vi "Acquire Triggered Images.vi"() -> ()   [LabVIEW 2023]
doc: "The Acquire Triggered Image example acquires images continuously and displays the images in an image control. This VI demonstrates how to configure a triggered acquisition using a grab."
uses:
  <vilib>/vision/driver/IMAQdx.llb/IMAQdx Buffer Number Mode.ctl
  <vilib>/vision/driver/NI_Vision_Acquisition_Software.lvlib
  <resource>/objmgr/imaqdx.rc
panel:
  out "Trigger Rate":dbl
  in  "Simulated Processing Delay (ms)":i32
  out "Images Behind":i32
  in  "Trigger Parameters":T1={"Trigger Mode"=0, "Trigger Activation"=0, "Timeout (ms)"=1000} {"Trigger Activation" items=["Rising Edge", "Falling Edge"]; "Trigger Mode" items=["Off", "On"]}
  in  "Camera Name":refnum<k21> caption="IMAQdx Session"
  out "Missed Trigger":bool
  out "Buffer Number":u32
  out "Image":T2(plugin-control)
  in  "Stop":bool
  # "Overview: Demonstrates how to dynamically enumerate the trigger modes and configure a triggered acquisition.\nRequirements: Vision Acquisition Software\nInstructions: \n1. Select the Camera Name\n2. Run the VI\n3. Select a Trigger Mode\n4. Specify a Timeout\n5. Increase the Simulated Processing Delay to see the effect on the Images Behind when the acquisition loop isn't executed as quickly as the camera acquires images."
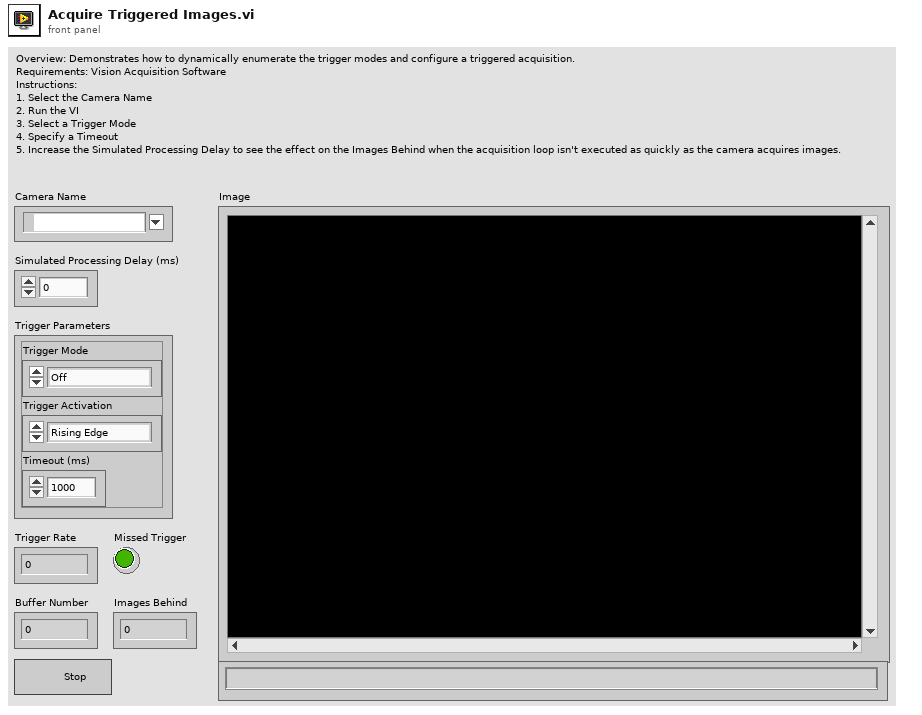
[diagram p1: front panel]
types:
  T1 = cluster{"Trigger Mode":u32, "Trigger Activation":u32, "Timeout (ms)":u32}
  T2 = typedef "IMAQ Image.ctl" = refnum<image>
  T3 = typedef "IMAQdx.ctl" = refnum<k21>
  T4 = typedef "NI_Vision_Acquisition_Software.lvlib/IMAQdx Buffer Number Mode.ctl" = enum32{"Next", "Last", "Buffer Number", "Every", "Last New"}
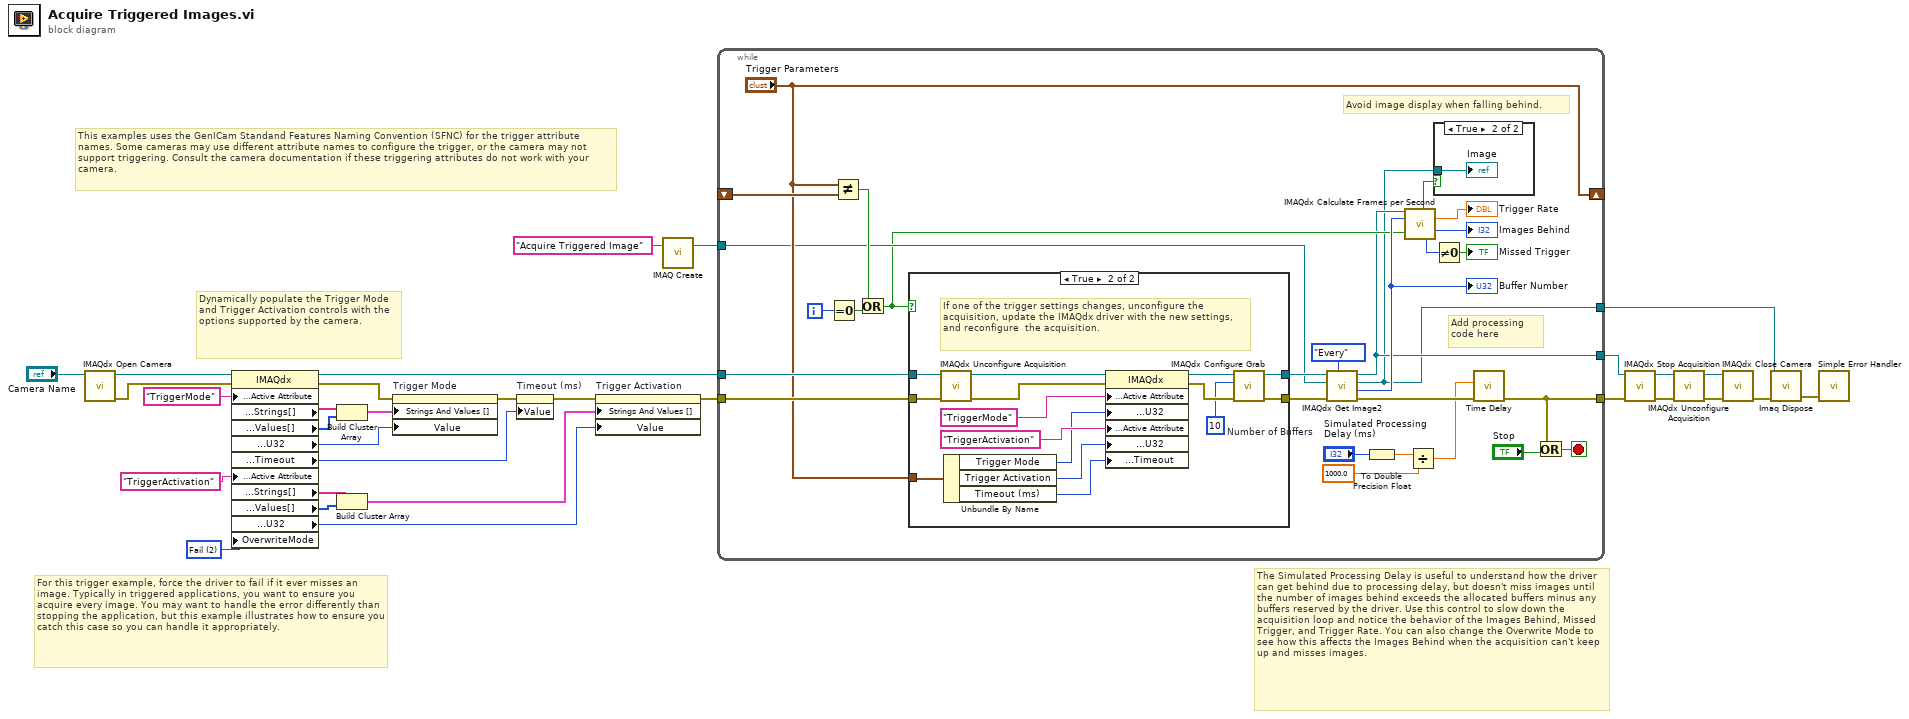
[diagram p0: block diagram]
diagram:
  w8 = u32 2 items=["Get Oldest"=0, "Fail"=2, "Get Newest"=3] ("OverwriteMode")
  # "The Simulated Processing Delay is useful to understand how the driver can get behind due to processing delay, but doesn't miss images until the number of images behind exceeds the allocated buffers minus any buffers reserved by the driver. Use this control to slow down the acquisition loop and notice the behavior of the Images Behind, Missed Trigger, and Trigger Rate. You can also change the Overwrite Mode to see how this affects the Images Behind when the acquisition can't keep up and misses images."
  # "For this trigger example, force the driver to fail if it ever misses an image. Typically in triggered applications, you want to ensure you acquire every image. You may want to handle the error differently than stopping the application, but this example illustrates how to ensure you catch this case so you can handle it appropriately."
  # "This examples uses the GenICam Standand Features Naming Convention (SFNC) for the trigger attribute names. Some cameras may use different attribute names to configure the trigger, or the camera may not support triggering. Consult the camera documentation if these triggering attributes do not work with your camera."
  # "Dynamically populate the Trigger Mode and Trigger Activation controls with the options supported by the camera."
  n1 = call <vilib>:"IMAQdx Open Camera.vi"("Session In"="Camera Name") -> ("error out"=w30:errorcluster, "Session Out"=w31:T3)  [unwired: 2 in, 7 out]
  n2 = property class="IMAQdx"(reference=w31, error in=w30, "Camera Attributes:Active Attribute"="TriggerMode" ("ActiveAttribute"), "Camera Attributes:Active Attribute"="TriggerActivation" ("ActiveAttribute"), "OverwriteMode"=w8) -> (reference out=w23:T3, error out=w25:errorcluster, "Camera Attributes:Enum:Strings[]"=w17:string[], "Camera Attributes:Enum:Values[]"=w16:u32[], "Camera Attributes:Value:U32"=w19:u32, "Acquisition Attributes:Timeout"=w22:u32, "Camera Attributes:Enum:Strings[]"=w14:string[], "Camera Attributes:Enum:Values[]"=w13:u32[], "Camera Attributes:Value:U32"=w18:u32)
  n3 = Build Cluster Array(w17, w16) -> (w15:cluster{string, u32}[])
  n4 = Build Cluster Array(w14, w13) -> (w12:cluster{string, u32}[])
  n5 = property on="Trigger Mode" class="Ring (strict)"(error in=w25, "Strings And Values []"=w15, "Value"=w19) -> (error out=w21:errorcluster)  [unwired: 1 in, 1 out]
  n6 = property on="Timeout (ms)" class="DigNum (strict)"(error in=w21, "Value"=w22) -> (error out=w20:errorcluster)  [unwired: 1 in, 1 out]
  n7 = property on="Trigger Activation" class="Ring (strict)"(error in=w20, "Strings And Values []"=w12, "Value"=w18) -> (error out=w24:errorcluster)  [unwired: 1 in, 1 out]
  n8 = call "IMAQ Create"("Image Name"="Acquire Triggered Image") -> ("New Image"=w27:T2)  [unwired: 3 in, 2 out]
  n9 = while {
    tunnel: [w44] -> w2
    tunnel: w23 -> [w57]
    tunnel: [w40] -> w3
    tunnel: w27 -> [w48]
    tunnel: w24 -> [w56]
    shift-right: ["Trigger Parameters"] -> _
    shift-left: _ -> [w55]
    tunnel: [w33] -> w10
    i -> [w54]
    stop <- w59 stop-if-true
    # "Avoid image display when falling behind."
    # "Add processing code here"
    n10 = Equal To 0?(x=w54) -> (x = 0?=w53:bool)
    n11 = Not Equal?(x="Trigger Parameters", y=w55) -> (x != y?=w52:bool)
    n12 = Or(x=w52, y=w53) -> (x .or. y?=w45:bool)
    n13 = case shown="True" w45 {
      tunnel: w57 -> [w62 w77]
      tunnel: [w62 w75] -> w50
      tunnel: w56 -> [w61 w76]
      tunnel: [w61 w74] -> w49
      tunnel: "Trigger Parameters" -> [_ w73]
      frame False {
      }
      frame True {
        w63 = u32 10  # Number of Buffers
        # "If one of the trigger settings changes, unconfigure the acquisition, update the IMAQdx driver with the new settings, and reconfigure  the acquisition."
        n14 = call <vilib>:"IMAQdx Unconfigure Acquisition.vi"("error in"=w76, "Session In"=w77) -> ("error out"=w71:errorcluster, "Session Out"=w72:T3)  [unwired: 8 out]
        n15 = Unbundle By Name(w73) -> ("Trigger Mode"=w66:u32, "Trigger Activation"=w65:u32, "Timeout (ms)"=w64:u32)
        n16 = property class="IMAQdx"(reference=w72, error in=w71, "Camera Attributes:Active Attribute"="TriggerMode" ("ActiveAttribute"), "Camera Attributes:Value:U32"=w66, "Camera Attributes:Active Attribute"="TriggerActivation" ("ActiveAttribute"), "Camera Attributes:Value:U32"=w65, "Acquisition Attributes:Timeout"=w64) -> (reference out=w70:T3, error out=w69:errorcluster)
        n17 = call <vilib>:"IMAQdx Configure Grab.vi"("error in"=w69, "Number of Buffers"=w63, "Session In"=w70) -> ("error out"=w74:errorcluster, "Session Out"=w75:T3)  [unwired: 7 out]
      }
    }
    n18 = call <vilib>:"IMAQdx Get Image2.vi"("Buffer Number Mode (Next)"=IMAQdx_Buffer_Number_Mode."Every", "error in"=w49, "Image In"=w48, "Session In"=w50) -> ("error out"=w41:errorcluster, "Buffer Number Out"=w46:u32, "Image Out"=w33:T2, "Session Out"=w44:T3)  [unwired: 4 in]
    "Buffer Number" <- w46
    n19 = To Double Precision Float(number="Simulated Processing Delay (ms)") -> (double precision float=w32:dbl)
    n20 = call <vilib>:"IMAQdx Calculate Frames per Second.vi"("Session In"=w44, "Buffer Number"=w46, "Reset Counters"=w45) -> ("Update Display"=w34:bool, "Acquired Frames per Second"=→"Trigger Rate":dbl, "Images Behind"=→"Images Behind":i32, "Images Missed"=w43:u32)  [unwired: 6 in, 3 out]
    n21 = Divide(x=w32, y=1000.0) -> (x/y=w36:dbl)
    n22 = case shown="True" w34 {
      tunnel: w33 -> [_ w60]
      frame False {
      }
      frame True {
        "Image" <- w60
      }
    }
    n23 = Not Equal To 0?(x=w43) -> (x != 0?=→"Missed Trigger":bool)
    n24 = call "Time Delay"("error in (no error)"=w41, "Delay Time (s)"=w36) -> ("error out"=w40:errorcluster)  [unwired: 9 in]
    n25 = Or(x=w40, y="Stop") -> (x .or. y?=w59:bool)
  }
  n26 = call <vilib>:"IMAQdx Stop Acquisition.vi"("error in"=w3, "Session In"=w2) -> ("error out"=w4:errorcluster, "Session Out"=w5:T3)  [unwired: 8 out]
  n27 = call <vilib>:"IMAQdx Unconfigure Acquisition.vi"("error in"=w4, "Session In"=w5) -> ("error out"=w7:errorcluster, "Session Out"=w6:T3)  [unwired: 8 out]
  n28 = call <vilib>:"IMAQdx Close Camera.vi"("error in"=w7, "Session In"=w6) -> ("error out"=w1:errorcluster)  [unwired: 9 out]
  n29 = call "Imaq Dispose"("Image"=w10, "error in (no error)"=w1) -> ("error out"=w9:errorcluster)  [unwired: 4 in]
  n30 = call <vilib>:"Simple Error Handler.vi"("error in (no error)"=w9) -> ()  [unwired: 1 in, 8 out]
